vi "DFD FXP NStage MRate Postprocessing (I32, 1Ch).vi"(5 "input range":dbl=1.0, 8 "error in (no error)":errorcluster, 10 "multirate filters":T1[](array[typedef]) {"mMRate_SumWl" min=1 max=32 step=1; "mMRate_InputIwl" min=1 max=32 step=1; "mMRate_GainWl" min=1 max=32 step=1; "mMRate_OutputWl" min=1 max=32 step=1; "mMRate_InputWl" min=1 max=32 step=1; "mMRate_CoefWl" min=1 max=32 step=1; "mMRate_Mode" items=["Default"=-1, "No Rate Change"=0, "Interpolation"=1, "Decimation"=2, "Interpolated"=3, "Rational"=4]}, 11 "signal in":i32[](array[numeric]) format="%.0x") -> (0 "error out":errorcluster, 3 "signal out":dbl[](array[numeric]))   [LabVIEW 2017, in "NI_DigFilterLicensed.lvlib"]
doc: "Converts the output signal of a fixed-point multistage multirate filter from a fixed-point representation to a floating-point representation. You must manually select the polymorphic instance you want to use."
uses:
  <vilib>/addons/Digital Filter Design/NI_DigFilterLicensed.lvlib
  <vilib>/addons/Digital Filter Design/_Objects.llb/DFD Multirate Filter Obj.ctl
  <vilib>/addons/Digital Filter Design/_Objects.llb/DFD Multirate Mode.ctl
  <vilib>/addons/Digital Filter Design/_Objects.llb/DFD Coef Norm Type.ctl
  <vilib>/addons/Digital Filter Design/_Objects.llb/DFD Round-off Mode.ctl
  <vilib>/addons/Digital Filter Design/_Objects.llb/DFD FXP MRate Multiply Mode.ctl
  <vilib>/addons/Digital Filter Design/_Misc.llb/dfd_Error Handlers (Single).vi
  <vilib>/addons/Digital Filter Design/NI_DigFilter_FXP.lvlib
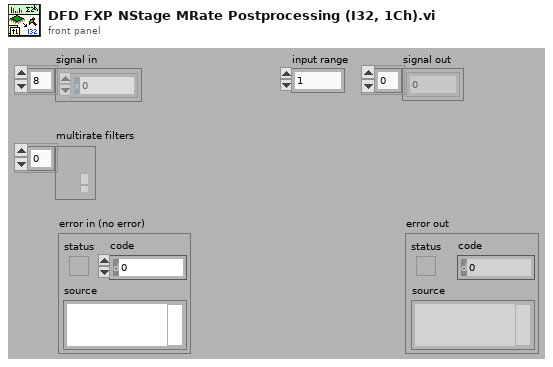
[diagram p1: front panel]
types:
  T1 = typedef "NI_DigFilterLicensed.lvlib/DFD Multirate Filter Obj.ctl" = cluster{"mMRate_Structure":enum16{"CIC", "FIR", "IIR", "Lattice"}, "mMRate_Mode":T2, "mMRate_Factor":i32, "mMRate_FIRParams":cluster{"mMRate_FIR_H":dbl[], "mMRate_FIR_IsNyquist?":bool, "mMRate_FIR_IsSymmetric?":bool}, "mMRate_CICParams":cluster{"mMRate_CIC_#Stage":i32, "mMRate_CIC_Lag":i32, "mMRate_CIC_Type":enum16{"Lowpass", "Highpass"}}, "mMRate_Order":i32, "mMRate_Version":string, "mMRate_Comments":string, "mMRate_RationalFactor":cluster{"mMRate_L":i32, "mMRate_M":i32}, "mMRate_Fs":dbl, "mMRate_Quantized?":bool, "mMRate_QFilterGain":dbl, "mMRate_CoefWl":i16, "mMRate_Scaling":cluster{"mMRate_ScaleByPowerOf2?":bool, "mMRate_ScaleType":T3}, "mMRate_InputWl":i16, "mMRate_OutputWl":i16, "mMRate_OutputMode":T4, "mMRate_MultMode":T5, "mMRate_BitPruning":bool, "mMRate_GainWl":i16, "mMRate_OutputFwl":i16, "mMRate_SumIwl":i16, "mMRate_InputIwl ":i16, "mMRate_SumWl":i16, "mMRate_CoefIwl":i16}
  T2 = typedef "NI_DigFilterLicensed.lvlib/DFD Multirate Mode.ctl" = i16
  T3 = typedef "NI_DigFilterLicensed.lvlib/DFD Coef Norm Type.ctl" = enum16{"No Norm", "Time Domain 1-Norm", "Time Domain 2-Norm", "Time Domain Inf-Norm"}
  T4 = typedef "NI_DigFilterLicensed.lvlib/DFD Round-off Mode.ctl" = enum16{"Nearest", "Truncation"}
  T5 = typedef "NI_DigFilterLicensed.lvlib/DFD FXP MRate Multiply Mode.ctl" = enum16{"Truncated", "Full"}
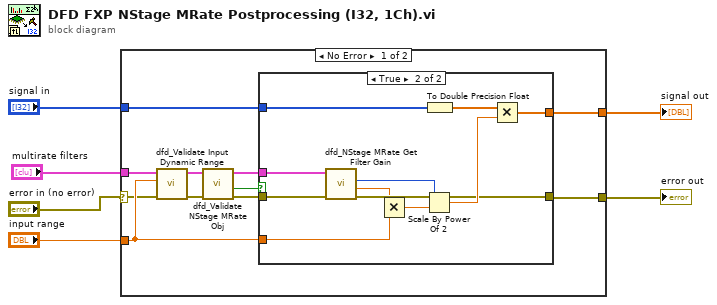
[diagram p0: block diagram]
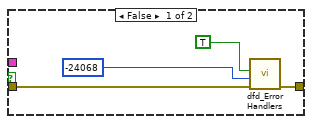
[diagram p2: hidden frame]
diagram:
  n1 = case shown="No Error" "error in (no error)" {
    selector: "error in (no error)" -> [w7 w31]
    tunnel: "signal in" -> [w16 _]
    tunnel: [w15 _] -> w5
    tunnel: [w13 w31] -> w4
    tunnel: "input range" -> [w11 _]
    tunnel: "multirate filters" -> [w10 _]
    frame No Error {
      n2 = call <vilib>:"dfd_Validate Input Dynamic Range.vi"("error in (no error)"=w7, "input range"=w11) -> ("error out"=w12:errorcluster)  [unwired: 9 out]
      n3 = call <vilib>:"dfd_Validate NStage MRate Obj.vi"("error in"=w12, "multirate filters"=w10) -> ("error out"=w8:errorcluster, "is valid FXP?"=w9:bool, "dup multirate filters"=w14:T1[])  [unwired: 7 out]
      n4 = case shown="True" w9 {
        tunnel: w11 -> [_ w30]
        tunnel: w16 -> [_ w26]
        tunnel: [_ w25] -> w15
        tunnel: w14 -> [_ w24]
        tunnel: w8 -> [w19 w23]
        tunnel: [w17 w23] -> w13
        frame False {
          n5 = call-poly <vilib>:"dfd_Error Handlers.vi"("error in (no error)"=w19, "error code"=-24068 ("ERR_INVALID_FXP_MRATE"), "condition failed?"=TRUE) -> ("error out"=w17:errorcluster)  [unwired: 8 out]
        }
        frame True {
          n6 = call <vilib>:"dfd_NStage MRate Get Filter Gain.vi"("multirate filters"=w24) -> ("gain"=w22:dbl, "NStage output -fwl"=w21:i16)  [unwired: 9 out]
          n7 = Multiply(x=w22, y=w30) -> (x*y=w29:dbl)
          n8 = Scale By Power Of 2(n=w21, x=w29) -> (x*2^n=w27:dbl)
          n9 = To Double Precision Float(number=w26) -> (double precision float=w28:dbl[])
          n10 = Multiply(x=w28, y=w27) -> (x*y=w25:dbl[])
        }
      }
    }
    frame Error {
    }
  }
  "signal out" <- w5
  "error out" <- w4
